vi "Cleanup.vi"(8 "error in (no error)":errorcluster, 11 "WebsocketStream in":refnum<class "WebsocketStream.lvclass">) -> (0 "error out":errorcluster)   [LabVIEW 2020, in "Stream-Websocket.lvlib" / "WebsocketStream.lvclass"]
uses:
  WebsocketStream.lvclass
  WebsocketStream.lvclass/WebsocketStream.ctl
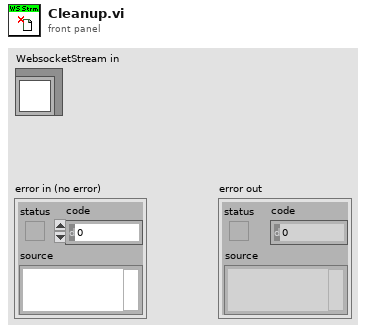
[diagram p1: front panel]
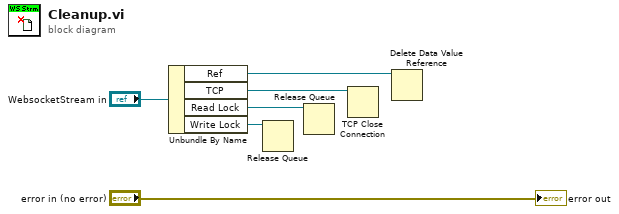
[diagram p0: block diagram]
diagram:
  n1 = Unbundle By Name("WebsocketStream in") -> ("Ref"=w1:refnum<data-value>, "TCP"=w2:refnum<k5>, "Read Lock"=w3:refnum<queue>, "Write Lock"=w4:refnum<queue>)
  n2 = Release Queue(queue=w4) -> ()  [unwired: 2 in, 3 out]
  n3 = Release Queue(queue=w3) -> ()  [unwired: 2 in, 3 out]
  n4 = TCP Close Connection(connection ID=w2) -> ()  [unwired: 2 in, 2 out]
  n5 = Delete Data Value Reference(data value reference=w1) -> ()  [unwired: 1 in, 2 out]
  "error out" <- "error in (no error)"
